vi "Write Misc Settings.vi"(4 "Section":string, 5 "error in (no error)":errorcluster, 6 "p_value":string, 7 "Key":string, 8 "Config Data in":refnum<class "Config Data.lvclass">) -> (0 "error out":errorcluster, 3 "Config Data out":refnum<class "Config Data.lvclass">)   [LabVIEW 2015, in "Config Data.lvlib" / "Config Data.lvclass"]
uses:
  Config Data.lvclass
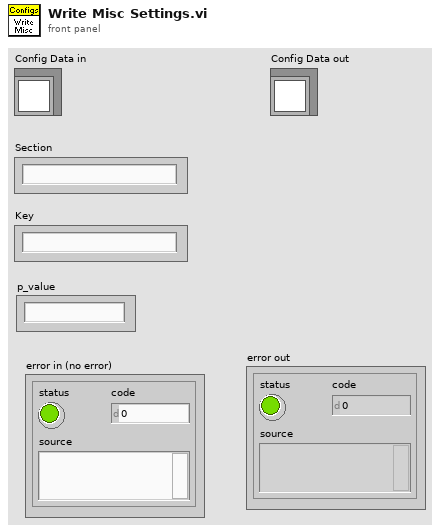
[diagram p1: front panel]
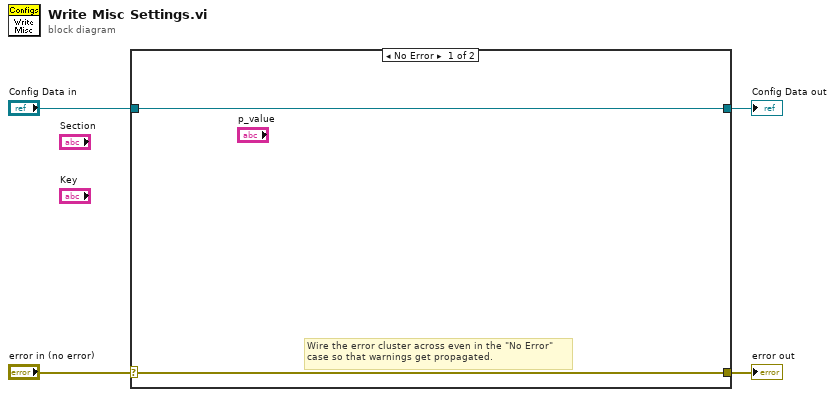
[diagram p0: block diagram]
diagram:
  n1 = case shown="No Error" "error in (no error)" {
    selector: "error in (no error)" -> [w5 w8]
    tunnel: [w5 w8] -> w3
    tunnel: [w6 w7] -> w1
    tunnel: "Config Data in" -> [w6 w7]
    frame No Error {
      # "Wire the error cluster across even in the \"No Error\"\ncase so that warnings get propagated."
    }
    frame Error {
    }
  }
  "error out" <- w3
  "Config Data out" <- w1
